vi "Customizing the Menubar.vi"() -> ()   [LabVIEW 2023]
doc: "This VI demonstrates how to programmatically add and remove items in a VI's run-time menubar."
uses:
  <vilib>/Utility/miscctls.llb/LVMenuShortCut.ctl
panel:
  in  "Remove Preferences":bool
  in  "Remove New":bool
  out "Selected Menu Item Tag":string
  in  "Stop":bool
  # "Overview: Demonstrates the use of the Menu functions to manipulate the contents of the run-time menubar of a VI.\nInstructions:\n1. Run the VI. Custom 'File' and 'Edit' menus will appear in the menubar.\n2. Select several different menu items. Those selections will be displayed in the Selected Menu Item Tag indicator.\n3. Click the two Remove buttons. Notice the 'File > New' and 'Edit > Preferences' menu items have been removed.\n4. Click Stop to stop the VI."
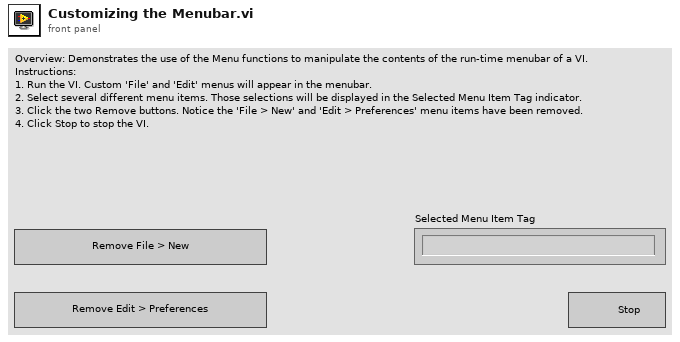
[diagram p1: front panel]
types:
  T1 = enum8{"Enabled", "Disabled", "Disabled and Grayed Out"}
  T2 = typedef "LVMenuShortCut.ctl" = cluster{"Include Shift Key?":bool, "Include Ctrl Key?":bool, "Shortcut Key":string}
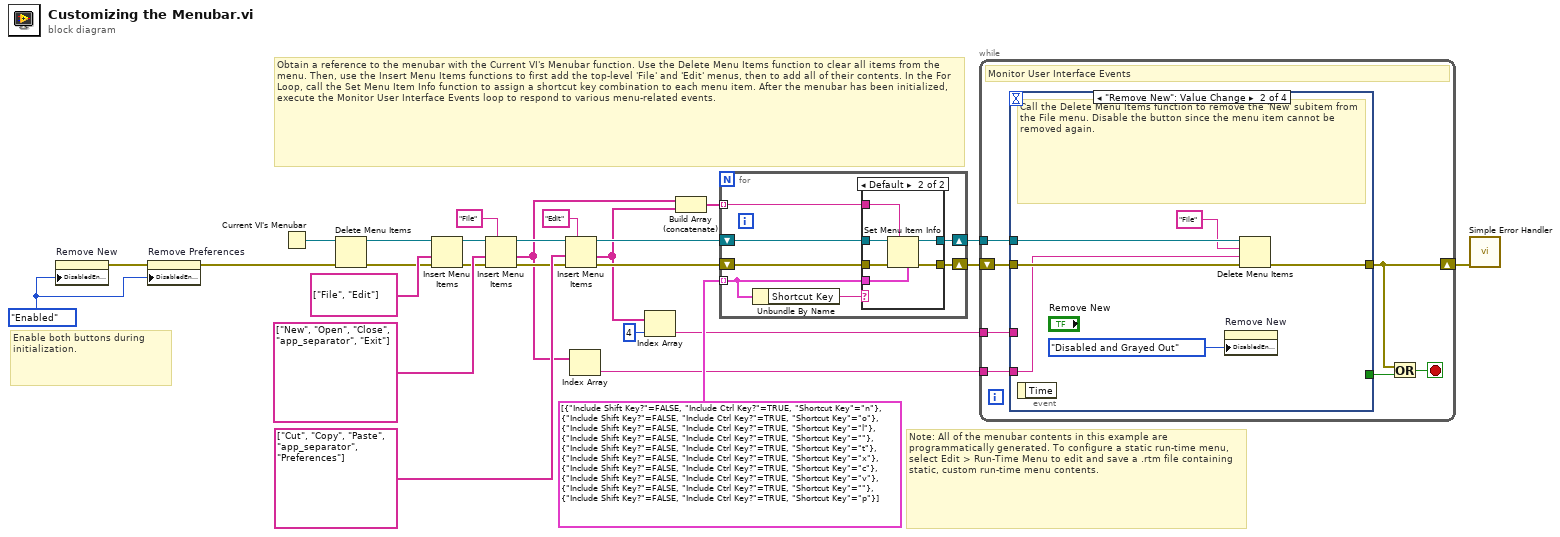
[diagram p0: block diagram]
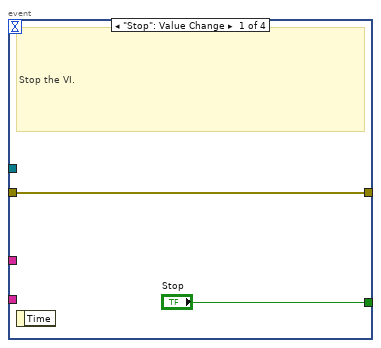
[diagram p2: hidden frame]
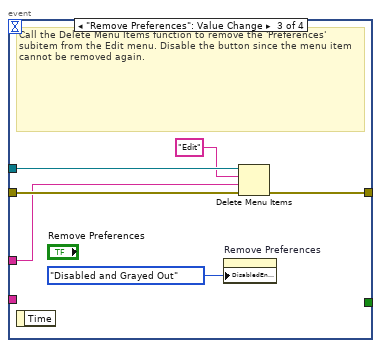
[diagram p3: hidden frame]
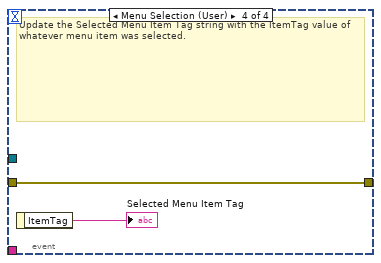
[diagram p4: hidden frame]
diagram:
  w1 = T1."Enabled" ("Disabled")
  # "Note: All of the menubar contents in this example are programmatically generated. To configure a static run-time menu, select Edit > Run-Time Menu to edit and save a .rtm file containing static, custom run-time menu contents."
  # "Enable both buttons during initialization."
  # "Obtain a reference to the menubar with the Current VI's Menubar function. Use the Delete Menu Items function to clear all items from the menu. Then, use the Insert Menu Items functions to first add the top-level 'File' and 'Edit' menus, then to add all of their contents. In the For Loop, call the Set Menu Item Info function to assign a shortcut key combination to each menu item. After the menubar has been initialized, execute the Monitor User Interface Events loop to respond to various menu-related events."
  n1 = property on="Remove New" class="Bool"("DisabledEnum"=w1) -> (error out=w3:errorcluster)  [unwired: 2 in, 1 out]
  n2 = property on="Remove Preferences" class="Bool"(error in=w3, "DisabledEnum"=w1) -> (error out=w2:errorcluster)  [unwired: 1 in, 1 out]
  n3 = Current VI's Menubar() -> (w17:refnum<k9>)
  n4 = Delete Menu Items(6:w2, 9:w17) -> (0:w12:errorcluster, 3:w18:refnum<k9>)  [unwired: 2 in]
  n5 = Insert Menu Items(6:w12, 7:string[] ["File", "Edit"] ("L10n_item tags 1"), 9:w18) -> (0:w16:errorcluster, 3:w27:refnum<k9>)  [unwired: 3 in, 1 out]
  n6 = Insert Menu Items(5:"File" ("L10n_menu tag"), 6:w16, 7:string[] ["New", "Open", "Close", "app_separator", "Exit"] ("L10n_item tags 2"), 9:w27) -> (0:w15:errorcluster, 1:w4:string[], 3:w26:refnum<k9>)  [unwired: 2 in]
  n7 = Insert Menu Items(5:"Edit" ("L10n_menu tag"), 6:w15, 7:string[] ["Cut", "Copy", "Paste", "app_separator", "Preferences"] ("L10n_item tags 3"), 9:w26) -> (0:w14:errorcluster, 1:w7:string[], 3:w25:refnum<k9>)  [unwired: 2 in]
  n8 = Index Array(array=w4) -> (element=w8:string)  [unwired: 1 in]
  n9 = Index Array(array=w7, index=4) -> (element=w6:string)
  n10 = Build Array (concatenate)(w4, w7) -> (w21:string[])
  n11 = for {
    tunnel: w21 -> [w33] mode=indexing
    tunnel: T2[] [{"Include Shift Key?"=FALSE, "Include Ctrl Key?"=TRUE, "Shortcut Key"="n"}, {"Include Shift Key?"=FALSE, "Include Ctrl Key?"=TRUE, "Shortcut Key"="o"}, {"Include Shift Key?"=FALSE, "Include Ctrl Key?"=TRUE, "Shortcut Key"="l"}, {"Include Shift Key?"=FALSE, "Include Ctrl Key?"=TRUE, "Shortcut Key"=""}, {"Include Shift Key?"=FALSE, "Include Ctrl Key?"=TRUE, "Shortcut Key"="t"}, {"Include Shift Key?"=FALSE, "Include Ctrl Key?"=TRUE, "Shortcut Key"="x"}, {"Include Shift Key?"=FALSE, "Include Ctrl Key?"=TRUE, "Shortcut Key"="c"}, {"Include Shift Key?"=FALSE, "Include Ctrl Key?"=TRUE, "Shortcut Key"="v"}, {"Include Shift Key?"=FALSE, "Include Ctrl Key?"=TRUE, "Shortcut Key"=""}, {"Include Shift Key?"=FALSE, "Include Ctrl Key?"=TRUE, "Shortcut Key"="p"}] -> [w29] mode=indexing
    shift-right: [w31] -> w13
    shift-left: w14 -> [w32]
    shift-right: [w30] -> w9
    shift-left: w25 -> [w34]
    n12 = Unbundle By Name(w29) -> ("Shortcut Key"=w28:string)
    n13 = case shown="Default" w28 {
      tunnel: w34 -> [w36 w42]
      tunnel: w33 -> [_ w41]
      tunnel: w32 -> [w35 w40]
      tunnel: [w35 w39] -> w31
      tunnel: [w36 w38] -> w30
      tunnel: w29 -> [_ w37]
      frame "" {
      }
      frame Default {
        n14 = Set Menu Item Info(4:w37, 7:w41, 8:w40, 11:w42) -> (0:w39:errorcluster, 3:w38:refnum<k9>)  [unwired: 3 in]
      }
    }
  }
  n15 = while {
    shift-right: [w46] -> w10
    shift-left: w13 -> [w49]
    tunnel: w9 -> [w45]
    tunnel: w8 -> [w44]
    tunnel: w6 -> [w43]
    stop <- w47 stop-if-true
    # "Monitor User Interface Events"
    n16 = event shown="[1] \"Remove New\": Value Change" {
      selector: _ -> [_ _ _ _]
      dyn-events: _ -> [_ _ _ _]
      timeout: _ -> [_ _ _ _]
      tunnel: w49 -> [w51 w56 w62 w64]
      tunnel: [w51 w57 w63 w64] -> w46
      tunnel: ["Stop" _ _ _] -> w48
      tunnel: w45 -> [_ w55 w61 _]
      tunnel: w44 -> [_ w53 _ _]
      tunnel: w43 -> [_ _ w59 _]
      event "Stop": Value Change {
        # "Stop the VI."
        n17 = event-data() -> ()  [unwired: 1 in, 1 out]
      }
      event "Remove New": Value Change {
        # "Call the Delete Menu Items function to remove the 'New' subitem from the File menu. Disable the button since the menu item cannot be removed again."
        n18 = event-data() -> ()  [unwired: 1 in, 1 out]
        n19 = property on="Remove New" class="Bool"("DisabledEnum"=T1."Disabled and Grayed Out" ("Disabled")) -> ()  [unwired: 2 in, 2 out]
        n20 = Delete Menu Items(6:w56, 7:w53, 8:"File" ("L10n_menu tag"), 9:w55) -> (0:w57:errorcluster)  [unwired: 1 out]
      }
      event "Remove Preferences": Value Change {
        # "Call the Delete Menu Items function to remove the 'Preferences' subitem from the Edit menu. Disable the button since the menu item cannot be removed again."
        n21 = event-data() -> ()  [unwired: 1 in, 1 out]
        n22 = property on="Remove Preferences" class="Bool"("DisabledEnum"=T1."Disabled and Grayed Out" ("Disabled")) -> ()  [unwired: 2 in, 2 out]
        n23 = Delete Menu Items(6:w62, 7:w59, 8:"Edit" ("L10n_menu tag"), 9:w61) -> (0:w63:errorcluster)  [unwired: 1 out]
      }
      event Menu Selection (User) {
        # "Update the Selected Menu Item Tag string with the ItemTag value of whatever menu item was selected."
        n24 = event-data() -> ("ItemTag"=→"Selected Menu Item Tag":string)  [unwired: 1 in]
      }
    }
    n25 = Or(x=w46, y=w48) -> (x .or. y?=w47:bool)
  }
  n26 = call <vilib>:"Simple Error Handler.vi"("error in (no error)"=w10) -> ()  [unwired: 4 in, 5 out]
